vi "ECA200.vi"() -> (1 "返回数":u32, 2 "读取缓冲区":string)   [LabVIEW 2020]
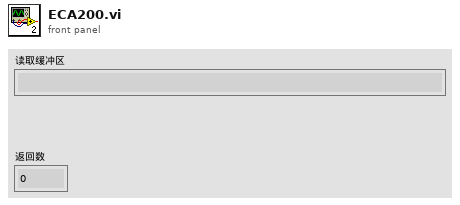
[diagram p1: front panel]
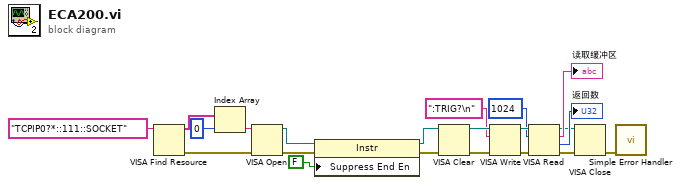
[diagram p0: block diagram]
diagram:
  n1 = VISA Find Resource(11:"TCPIP0?*::111::SOCKET" ("表达式(\"?*\")")) -> (0:w1:errorcluster, 3:w8:string[])  [unwired: 2 in, 1 out]
  n2 = Index Array(array=w8, index=0 ("索引")) -> (element=w6:string)
  n3 = VISA Open(error in (no error)=w1, VISA resource name=w6) -> (VISA resource name=w3:refnum<visa-resource-name>, error out=w2:errorcluster)  [unwired: 3 in]
  n4 = property class="Instr"(reference=w3, error in=w2, "Suppress End En"=FALSE ("Message Based Settings:Suppress End Enable")) -> (reference out=w5:refnum<visa-resource-name>, error out=w4:errorcluster)
  n5 = VISA Clear(VISA resource name=w5, error in (no error)=w4) -> (VISA resource name out=w21:refnum<visa-resource-name>, error out=w20:errorcluster)
  n6 = VISA Write(VISA resource name=w21, write buffer=":TRIG?\n" ("写入缓冲区"), error in (no error)=w20) -> (VISA resource name out=w18:refnum<visa-resource-name>, error out=w17:errorcluster)  [unwired: 1 out]
  n7 = VISA Read(VISA resource name=w18, byte count=u32 1024 ("字节总数"), error in (no error)=w17) -> (VISA resource name out=w12:refnum<visa-resource-name>, read buffer=→"读取缓冲区":string, return count=→"返回数":u32, error out=w11:errorcluster)
  n8 = VISA Close(VISA resource name=w12, error in (no error)=w11) -> (error out=w10:errorcluster)
  n9 = call <vilib>:"Simple Error Handler.vi"("error in (no error)"=w10) -> ()  [unwired: 4 in, 5 out]
